vi "Util_Trajectory_ReadFile.vi"(8 "error in (no error)":errorcluster, 11 "FileName":string="trajectory.csv") -> (0 "error out":errorcluster, 3 "outTRAJECTORY":T1 {"States"."POSE"."ROTATION"."SIN" format="%13.4f"; "States"."POSE"."ROTATION"."COS" format="%13.4f"; "States"."POSE"."ROTATION"."VALUE" format="%13.4f"; "States"."POSE"."TRANSLATION"."Y" format="%14.3f"; "States"."POSE"."TRANSLATION"."X" format="%14.3f"; "TotalTImeSecs" format="%20.3f"}, 4 "Full FIlename":string)   [LabVIEW 2019, in "Trajectory_Library.lvlib"]
doc: "Create a trajectory from a CSV file. This can be used on a PC or the RoboRIO. Normally the CSV file is created as output from one of the trajectory utility programs. The file could also be created manually or by a custom written program.\n\nParameters:\n - FileName -- Name of the CSV file to read. See file name notes for additional information.\n - Error In -- Input error cluster (optional)\n\nReturns:\n - outTrajectory - Trajectory data structure cluster\n - Error out - returned error cluster\n\nNotes on use:\n -- This routine writes informational messges to the console and to the driver station log.\n\nNotes on file naming:\n -- The file name must include the extention. \".csv\" is not automatically appended to the name. \n -- The file name can be a simple file or an absolute path. If a simple file name is used the default path on the RoboRIO is: \"home:\\lvuser\\natinst\\LabVIEW Data\". On a Windows PC the default path is the LabVIEW default directory. Normally this is: “%HOMEDRIVE%%HOMEPATH%\\Documents\\LabView Data\".\n -- Filenames on the RoboRIO, which runs Linux, are case sensitive.\n\nNotes on file contents:\n -- Blank lines are ignored.\n -- Lines that begin with either #, !, or ' in the first character are considered comments and are ignored. \n -- Other lines are interpretted as comma separated data as follows:\n -- Trajectory time -- seconds\n -- Expected velocity -- meters/sec\n -- Expected acceleration -- meters/sec^2\n -- Expected X position -- meters\n -- Expected Y position -- meters\n -- Expected heading (not necessarily robot orientation) -- radians\n -- Expected curvature (rotational portion of velocity) -- radians/meter\n -- Optional comment string. This ignored when reading file"
uses:
  Trajectory_Library.lvlib
  TypeDef/TRAJECTORY.ctl
  TypeDef/TRAJ_STATE.ctl
  TypeDef/POSE2D.ctl
  TypeDef/TRANSLATION2D.ctl
  TypeDef/ROTATION2D.ctl
  <vilib>/Utility/error.llb/whitespace.ctl
  Rotation2d_CreateAngle.vi
  Translation2d_Create.vi
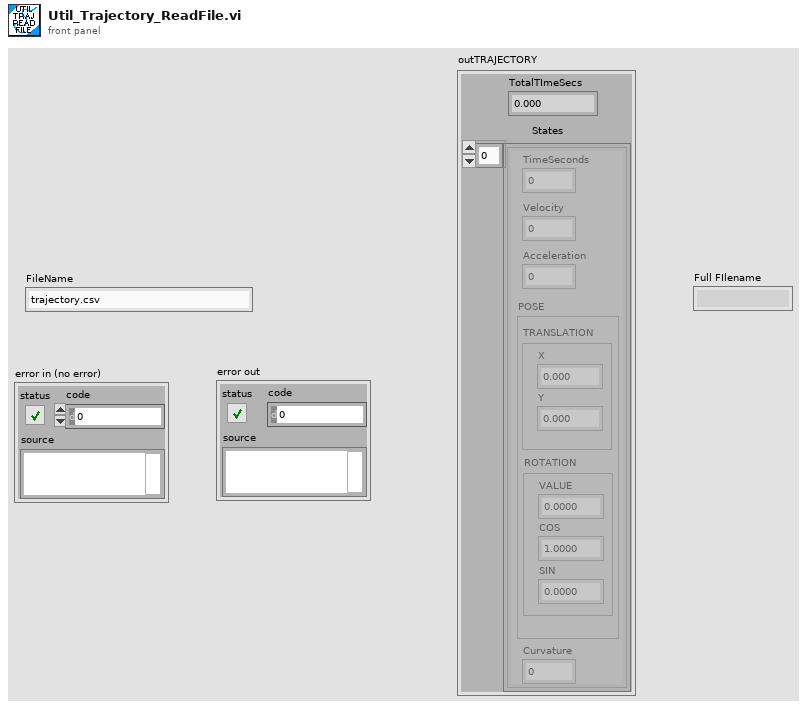
[diagram p1: front panel]
types:
  T1 = typedef "Trajectory_Library.lvlib/TRAJECTORY.ctl" = cluster{"TotalTImeSecs":dbl, "States":T2[]}
  T2 = typedef "Trajectory_Library.lvlib/TRAJ_STATE.ctl" = cluster{"TimeSeconds":dbl, "Velocity":dbl, "Acceleration":dbl, "POSE":T3, "Curvature":dbl}
  T3 = typedef "Trajectory_Library.lvlib/POSE2D.ctl" = cluster{"TRANSLATION":T4, "ROTATION":T5}
  T4 = typedef "Trajectory_Library.lvlib/TRANSLATION2D.ctl" = cluster{"X":dbl, "Y":dbl}
  T5 = typedef "Trajectory_Library.lvlib/ROTATION2D.ctl" = cluster{"VALUE":dbl, "COS":dbl, "SIN":dbl}
  T6 = enum16{"open", "replace", "create", "open or create", "replace or create", "replace or create with confirmation"}
  T7 = typedef "whitespace.ctl" = u16
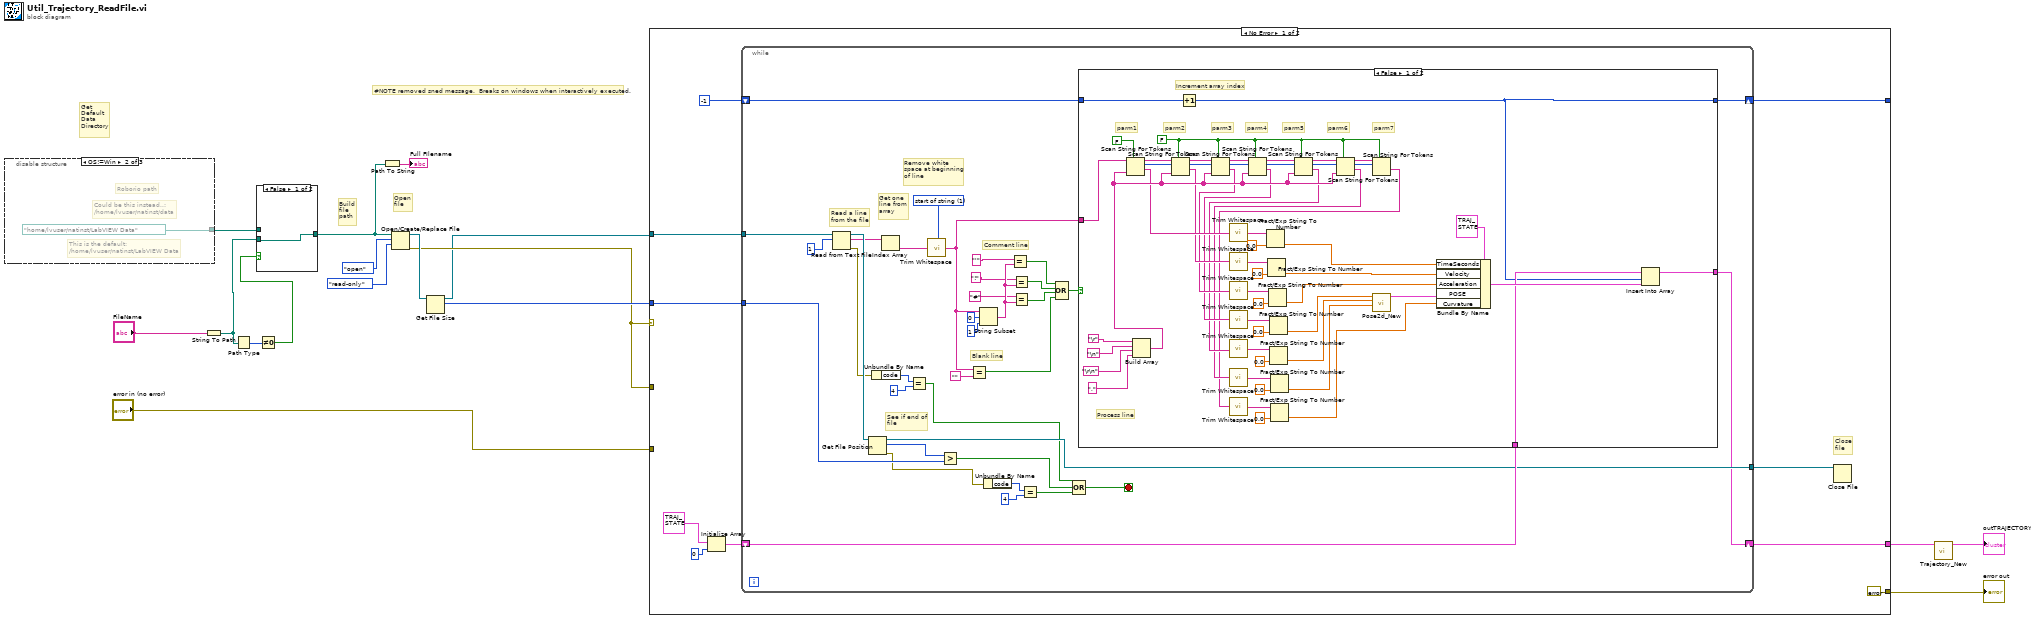
[diagram p0: block diagram]
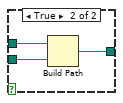
[diagram p2: hidden frame]
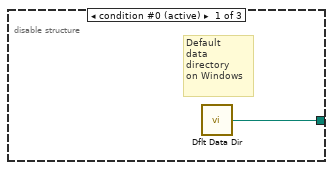
[diagram p3: hidden frame]
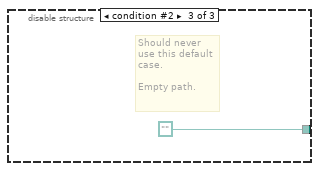
[diagram p4: hidden frame]
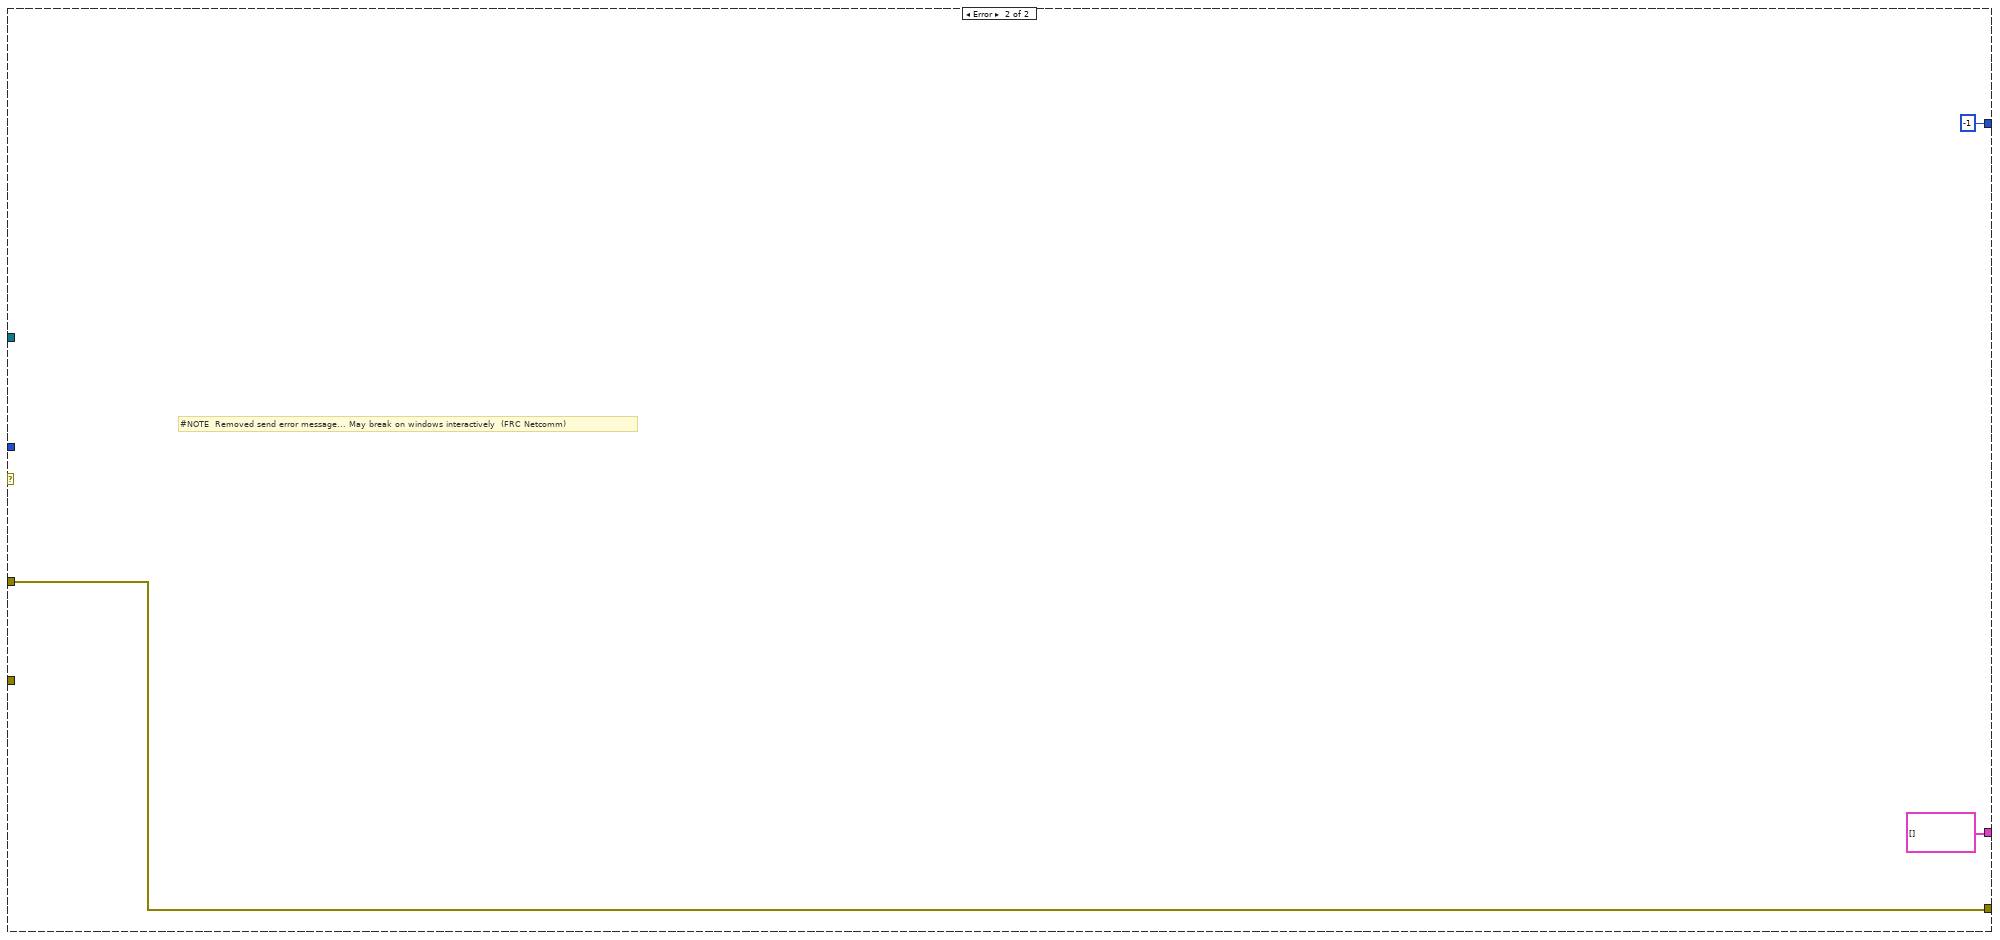
[diagram p6: hidden frame]
diagram:
  # "#NOTE removed sned message.  Breaks on windows when interactively executed."
  # "Get\nDefault\nData\nDirectory"
  # "Open\nfile"
  # "Build\nfile\npath"
  n1 = disable-structure shown="OS!=Win" {
    disable-tunnel: [w18 path "/home/lvuser/natinst/LabVIEW Data" path ""] -> w11
    frame condition #0 (active) {
      # "Default\ndata\ndirectory\non Windows"
      n2 = call <vilib>:"Dflt Data Dir.vi"() -> ("App:Default Data Directory"=w18:path)
    }
    frame condition #1 {
      # "This is the default:\n/home/lvuser/natinst/LabVIEW Data"
      # "Could be this instead..:\n/home/lvuser/natinst/data"
      # "Roborio path"
    }
    frame condition #2 {
      # "Should never\nuse this default\ncase.\n\nEmpty path."
    }
  }
  n3 = String To Path(string="FileName") -> (path=w6:path)
  n4 = Path Type(1:w6) -> (0:w5:i16)
  n5 = Not Equal To 0?(x=w5) -> (x != 0?=w4:bool)
  n6 = case shown="False" w4 {
    tunnel: [w21 w24] -> w14
    tunnel: w11 -> [_ w23]
    tunnel: w6 -> [w21 w22]
    frame False {
    }
    frame True {
      n7 = Build Path(base path=w23, name or relative path=w22) -> (appended path=w24:path)
    }
  }
  n8 = Path To String(path=w14) -> (string=→"Full FIlename":string)
  n9 = Open/Create/Replace File(file path (use dialog)=w14, operation (0:open)=T6."open", access (0:read/write)=enum16{"read/write", "read-only", "write-only"}."read-only") -> (refnum out=w15:refnum<file>, error out=w12:errorcluster)  [unwired: 3 in, 1 out]
  n10 = Get File Size(file=w15) -> (refnum out=w3:refnum<file>, size (in bytes)=w13:i64)  [unwired: 1 in, 1 out]
  n11 = case shown="No Error" w12 {
    tunnel: w3 -> [w34 _]
    tunnel: w13 -> [w32 _]
    tunnel: [w28 i16 -1] -> _
    tunnel: [w27 T2[] []] -> w10
    tunnel: w12 -> [_ w128]
    tunnel: [errorcluster {"status"=FALSE, "code"=0, "source"=""} ("error out") w128] -> w8
    tunnel: "error in (no error)" -> [_ _]
    frame No Error {
      # "Close\nfile"
      n12 = Initialize Array(T2 {"TimeSeconds"=0.0, "Velocity"=0.0, "Acceleration"=0.0, "POSE"={"TRANSLATION"={"X"=0.0, "Y"=0.0}, "ROTATION"={"VALUE"=0.0, "COS"=1.0, "SIN"=0.0}}, "Curvature"=0.0} ("TRAJ_STATE"), 0 ("dimension size")) -> (w29:T2[])
      n13 = while {
        tunnel: w34 -> [w70]
        tunnel: w32 -> [w66]
        tunnel: [w46] -> w31
        shift-right: [w36] -> w28
        shift-left: i16 -1 -> [w50]
        shift-right: [w35] -> w27
        shift-left: w29 -> [w48]
        stop <- w44 stop-if-true
        w65 = T7 1 items=["both", "start of string", "end of string"] ("location (both)")
        # "Comment line"
        # "Blank line"
        # "Remove white \nspace at beginning\nof line"
        # "Get one\nline from\narray"
        # "Read a line\nfrom the file"
        # "See if end of \nfile"
        n14 = Read from Text File(file (use dialog)=w70, count=1) -> (refnum out=w68:refnum<file>, text=w64:string[], error out=w47:errorcluster)  [unwired: 2 in, 1 out]
        n15 = Get File Position(7:w68) -> (0:w39:errorcluster, 2:w67:i64, 3:w46:refnum<file>)  [unwired: 1 in]
        n16 = Unbundle By Name(w47) -> ("code"=w43:i32)
        n17 = Index Array(array=w64) -> (element=w63:string)  [unwired: 1 in]
        n18 = Equal?(x=w43, y=4) -> (x = y?=w38:bool)
        n19 = call <vilib>:"Trim Whitespace.vi"("string"=w63, "location (both)"=w65) -> ("trimmed string"=w49:string)
        n20 = Greater?(x=w67, y=w66) -> (0:w45:bool)
        n21 = Equal?(x=w49, y="") -> (x = y?=w52:bool)
        n22 = String Subset(string=w49, offset (0)=0, length (rest)=1 ("length (rest)")) -> (substring=w59:string)
        n23 = Unbundle By Name(w39) -> ("code"=w41:i32)
        n24 = Equal?(x="'", y=w59) -> (x = y?=w55:bool)
        n25 = Equal?(x="!", y=w59) -> (x = y?=w54:bool)
        n26 = Equal?(x="#", y=w59) -> (x = y?=w53:bool)
        n27 = Equal?(x=w41, y=4) -> (x = y?=w37:bool)
        n28 = Compound Arithmetic op=OR(w55, w54, w53, w52) -> (w51:bool)
        n29 = Compound Arithmetic op=OR(w38, w45, w37) -> (w44:bool)
        n30 = case shown="False" w51 {
          tunnel: w50 -> [w125 w126]
          tunnel: [w88 w126] -> w36
          tunnel: w49 -> [w87 _]
          tunnel: w48 -> [w90 w127]
          tunnel: [w89 w127] -> w35
          frame False {
            w77 = FALSE ("allow empty tokens? (F)")
            # "parm6"
            # "parm7"
            # "parm5"
            # "parm4"
            # "parm3"
            # "parm2"
            # "parm1"
            # "Increment array index"
            # "Process line"
            n31 = Build Array("\r", "\n", "\r\n", ",") -> (w119:string[])
            n32 = Scan String For Tokens(5:FALSE ("allow empty tokens? (F)"), 6:w119, 9:w87) -> (1:w108:string, 2:w113:i32, 3:w118:string)  [unwired: 3 in, 1 out]
            n33 = Scan String For Tokens(5:w77, 6:w119, 8:w113, 9:w118) -> (1:w107:string, 2:w112:i32, 3:w117:string)  [unwired: 2 in, 1 out]
            n34 = Increment(x=w125) -> (x+1=w88:i16)
            n35 = Scan String For Tokens(5:w77, 6:w119, 8:w112, 9:w117) -> (1:w106:string, 2:w111:i32, 3:w116:string)  [unwired: 2 in, 1 out]
            n36 = call <vilib>:"Trim Whitespace.vi"("string"=w108) -> ("trimmed string"=w72:string)  [unwired: 1 in]
            n37 = call <vilib>:"Trim Whitespace.vi"("string"=w107) -> ("trimmed string"=w101:string)  [unwired: 1 in]
            n38 = call <vilib>:"Trim Whitespace.vi"("string"=w106) -> ("trimmed string"=w96:string)  [unwired: 1 in]
            n39 = Scan String For Tokens(5:w77, 6:w119, 8:w111, 9:w116) -> (1:w105:string, 2:w110:i32, 3:w115:string)  [unwired: 2 in, 1 out]
            n40 = call <vilib>:"Trim Whitespace.vi"("string"=w105) -> ("trimmed string"=w95:string)  [unwired: 1 in]
            n41 = Fract/Exp String To Number(string=w72, default (0 dbl)=0.0 ("default (0 DBL)")) -> (number=w73:dbl)  [unwired: 2 in, 1 out]
            n42 = Fract/Exp String To Number(string=w101, default (0 dbl)=0.0 ("default (0 DBL)")) -> (number=w92:dbl)  [unwired: 2 in, 1 out]
            n43 = Fract/Exp String To Number(string=w96, default (0 dbl)=0.0 ("default (0 DBL)")) -> (number=w85:dbl)  [unwired: 2 in, 1 out]
            n44 = Fract/Exp String To Number(string=w95, default (0 dbl)=0.0 ("default (0 DBL)")) -> (number=w83:dbl)  [unwired: 2 in, 1 out]
            n45 = Scan String For Tokens(5:w77, 6:w119, 8:w110, 9:w115) -> (1:w104:string, 2:w109:i32, 3:w114:string)  [unwired: 2 in, 1 out]
            n46 = call <vilib>:"Trim Whitespace.vi"("string"=w104) -> ("trimmed string"=w94:string)  [unwired: 1 in]
            n47 = Fract/Exp String To Number(string=w94, default (0 dbl)=0.0 ("default (0 DBL)")) -> (number=w82:dbl)  [unwired: 2 in, 1 out]
            n48 = Scan String For Tokens(5:w77, 6:w119, 8:w109, 9:w114) -> (1:w103:string, 2:w75:i32, 3:w76:string)  [unwired: 2 in, 1 out]
            n49 = call <vilib>:"Trim Whitespace.vi"("string"=w103) -> ("trimmed string"=w93:string)  [unwired: 1 in]
            n50 = Fract/Exp String To Number(string=w93, default (0 dbl)=0.0 ("default (0 DBL)")) -> (number=w81:dbl)  [unwired: 2 in, 1 out]
            n51 = Scan String For Tokens(5:w77, 8:w75, 9:w76) -> (1:w74:string)  [unwired: 3 in, 3 out]
            n52 = call <vilib>:"Trim Whitespace.vi"("string"=w74) -> ("trimmed string"=w79:string)  [unwired: 1 in]
            n53 = Fract/Exp String To Number(string=w79, default (0 dbl)=0.0 ("default (0 DBL)")) -> (number=w78:dbl)  [unwired: 2 in, 1 out]
            n54 = call "Pose2d_New.vi"("Heading"=w81, "Y"=w82, "X"=w83) -> ("out POSe"=w84:T3)  [unwired: 8 in]
            n55 = Bundle By Name(cluster=T2 {"TimeSeconds"=0.0, "Velocity"=0.0, "Acceleration"=0.0, "POSE"={"TRANSLATION"={"X"=0.0, "Y"=0.0}, "ROTATION"={"VALUE"=0.0, "COS"=1.0, "SIN"=0.0}}, "Curvature"=0.0} ("TRAJ_STATE"), "TimeSeconds"=w73, "Velocity"=w92, "Acceleration"=w85, "POSE"=w84, "Curvature"=w78) -> (w91:T2)
            n56 = Insert Into Array(array=w90, index=w88, new element=w91) -> (w89:T2[])
          }
          frame True {
            # "Comment -- ignore."
          }
        }
      }
      n57 = Close File(refnum=w31) -> ()  [unwired: 1 in, 2 out]
    }
    frame Error {
      # "#NOTE  Removed send error message... May break on windows interactively  (FRC Netcomm)"
    }
  }
  "error out" <- w8
  n58 = call "Trajectory_New.vi"("TRAJ_STATES"=w10) -> ("TRAJECTORY"=→"outTRAJECTORY":T1)  [unwired: 10 in]
